vi "Handle Messages.vi"(8 "error in (no error)":errorcluster, 9 "Message Data":variant, 10 "Message":string, 11 "Coffee Shop In":refnum<class "Coffee Shop.lvclass">) -> (0 "error out":errorcluster, 3 "Coffee Shop Out":refnum<class "Coffee Shop.lvclass">)   [LabVIEW 2020, in "Coffee Shop.lvclass"]
uses:
  Coffee Shop.lvclass
  C:/Program Files (x86)/National Instruments/LabVIEW 2020/vi.lib/Asteme/Triarc Framework/Application/Application.lvclass
  C:/Program Files (x86)/National Instruments/LabVIEW 2020/vi.lib/Asteme/Triarc Framework/Process/Process.lvclass
  Customer/Customer.lvclass
  Public/Roles.ctl
  <vilib>/Asteme/Triarc Framework/Process/Process.lvclass/Process.ctl
  <vilib>/Asteme/Triarc Framework/Application/Application.lvclass/Application.ctl
  Coffee Shop.lvclass/Coffee Shop.ctl
  Process Job/Job Handler.lvclass
  <vilib>/Asteme/Triarc Framework/Application/Private/Add Process to Map.vi
  <vilib>/Asteme/Triarc Framework/Application/Private/Start Idle Processes if Running.vi
  <vilib>/Asteme/Triarc Framework/Process/Protected/Messaging/Enqueue Message.vi
  <vilib>/Asteme/Triarc Framework/Process/Protected/SubVIs/Set Context.vi
  <vilib>/Asteme/Triarc Framework/Process/Public/Lifecycle/Get Lifecycle State.vi
  <vilib>/Asteme/Triarc Framework/Process/Stop.vi
  <vilib>/Utility/error.llb/Clear Errors.vi
  <vilib>/Asteme/Triarc Framework/Process/Community/Leave Process Loop.vi
  <vilib>/Asteme/Triarc Framework/Process/Private/SubVIs/Wait for finish.vi
  <vilib>/Asteme/Triarc Framework/Process/Private/SubVIs/Set Lifecycle State.vi
  <vilib>/Asteme/Triarc Framework/Application/Application.lvclass
  <vilib>/Utility/error.llb/Error Cluster From Error Code.vi
  <vilib>/Asteme/Triarc Framework/Process/Start.vi
  <vilib>/Asteme/Triarc Framework/Application/Private/Update Context for Owned Processes.vi
  <vilib>/Asteme/Triarc Framework/Process/Process.lvclass
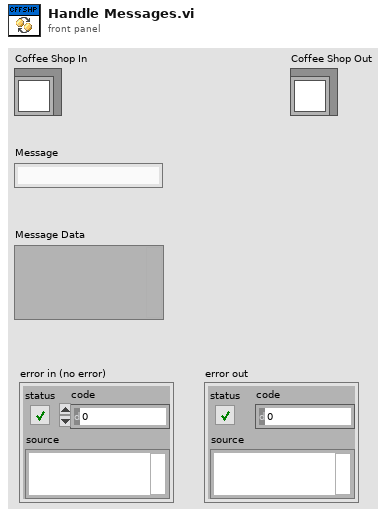
[diagram p1: front panel]
types:
  T1 = typedef "Coffee Shop.lvclass/Roles.ctl" = enum16{"Customer", "Barista", "Cashier"}
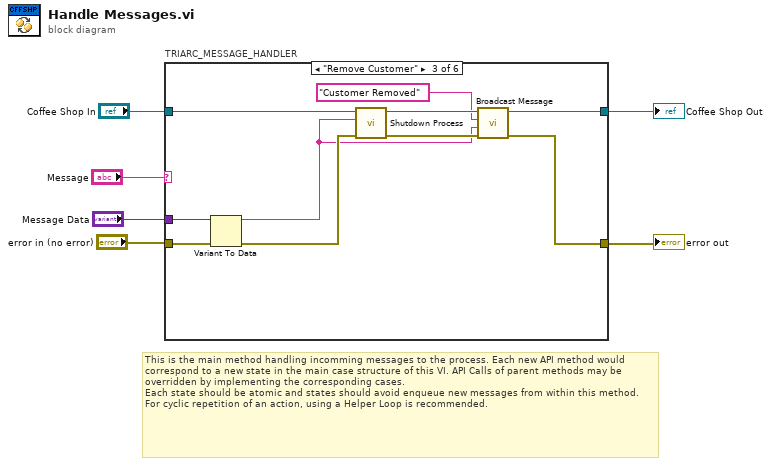
[diagram p0: block diagram]
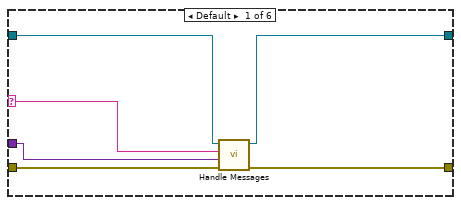
[diagram p2: hidden frame]
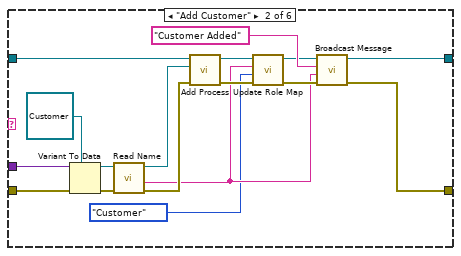
[diagram p3: hidden frame]
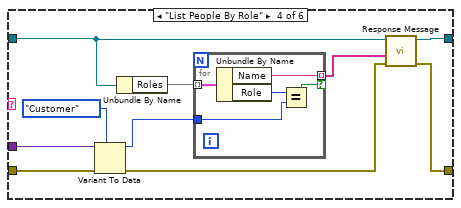
[diagram p4: hidden frame]
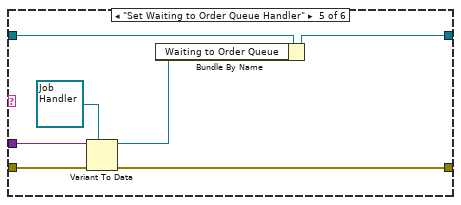
[diagram p5: hidden frame]
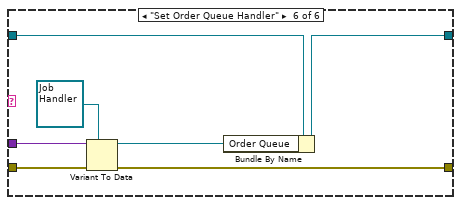
[diagram p6: hidden frame]
diagram:
  # "This is the main method handling incomming messages to the process. Each new API method would correspond to a new state in the main case structure of this VI. API Calls of parent methods may be overridden by implementing the corresponding cases.\nEach state should be atomic and states should avoid enqueue new messages from within this method. For cyclic repetition of an action, using a Helper Loop is recommended."
  n1 = case "TRIARC_MESSAGE_HANDLER" shown="\"Remove Customer\"" "Message" {
    selector: "Message" -> [w10 _ _ _ _ _]
    tunnel: "error in (no error)" -> [w9 w28 w39 w49 w61 w68]
    tunnel: "Coffee Shop In" -> [w12 w26 w37 w41 w60 w67]
    tunnel: "Message Data" -> [w11 w29 w38 w47 w57 w64]
    tunnel: [w8 w23 w34 w43 w59 w66] -> w2
    tunnel: [w7 w22 w32 w42 w56 w63] -> w1
    frame Default {
      n2 = call-parent "Handle Messages.vi"("error in (no error)"=w9, "Message Data"=w11, "Message"=w10, "Application In"=w12) -> ("error out"=w8:errorcluster, "Application Out"=w7:refnum<class "Coffee Shop.lvclass">)  [unwired: 6 in]
    }
    frame "Add Customer" {
      n3 = Variant To Data(error in=w28, type=refnum<class "Customer.lvclass"> refnum ("Customer.lvclass"), Variant=w29) -> (data=w19:refnum<class "Customer.lvclass">, error out=w25:errorcluster)
      n4 = call-dynamic "Read Name.vi"("error in (no error)"=w25, "Process In"=w19) -> ("error out"=w20:errorcluster, "Name"=w14:string, "Process Out"=w18:refnum<class "Customer.lvclass">)  [unwired: 6 in, 1 out]
      n5 = call <vilib>:"Add Process.vi"("error in (no error)"=w20, "Process"=w18, "Rig In"=w26) -> ("error out"=w24:errorcluster, "Rig Out"=w16:refnum<class "Coffee Shop.lvclass">)  [unwired: 7 in]
      n6 = call "Update Role Map.vi"("error in (no error)"=w24, "Role"=Roles."Customer", "Name"=w14, "Coffee Shop In"=w16) -> ("error out"=w17:errorcluster, "Coffee Shop Out"=w15:refnum<class "Coffee Shop.lvclass">)  [unwired: 6 in]
      n7 = call-dynamic "Broadcast Message.vi"("error in (no error)"=w17, "Message Data"=w14, "Message"="Customer Added", "Rig Process In"=w15) -> ("error out"=w23:errorcluster, "Rig Process Out"=w22:refnum<class "Coffee Shop.lvclass">)  [unwired: 6 in]
    }
    frame "Remove Customer" {
      n8 = Variant To Data(error in=w39, Variant=w38) -> (data=w30:string, error out=w36:errorcluster)  [unwired: 1 in]
      n9 = call <vilib>:"Shutdown Process.vi"("error in (no error)"=w36, "Process Name"=w30, "Rig In"=w37) -> ("error out"=w35:errorcluster, "Rig Out"=w33:refnum<class "Coffee Shop.lvclass">)  [unwired: 7 in]
      n10 = call-dynamic "Broadcast Message.vi"("error in (no error)"=w35, "Message Data"=w30, "Message"="Customer Removed", "Rig Process In"=w33) -> ("error out"=w34:errorcluster, "Rig Process Out"=w32:refnum<class "Coffee Shop.lvclass">)  [unwired: 6 in]
    }
    frame "List People By Role" {
      n11 = Variant To Data(error in=w49, type=Roles."Customer" ("Roles"), Variant=w47) -> (data=w44:T1, error out=w48:errorcluster)
      n12 = Unbundle By Name(w41) -> ("Roles"=w45:map{string, T1})
      n13 = for {
        tunnel: w45 -> [w54] mode=indexing
        tunnel: w44 -> [w50]
        tunnel: [w53] -> w40 mode=indexing if=w52
        n14 = Unbundle By Name(w54) -> ("Name"=w53:string, "Role"=w51:T1)
        n15 = Equal?(x=w51, y=w50) -> (x = y?=w52:bool)
      }
      n16 = call <vilib>:"Response Message.vi"("error in (no error)"=w48, "Response Message Data"=w40, "Process In"=w41) -> ("error out"=w43:errorcluster, "Process Out"=w42:refnum<class "Coffee Shop.lvclass">)  [unwired: 7 in]
    }
    frame "Set Waiting to Order Queue Handler" {
      n17 = Variant To Data(error in=w61, type=refnum<class "Job Handler.lvclass"> refnum ("Job Handler.lvclass"), Variant=w57) -> (data=w55:refnum<class "Job Handler.lvclass">, error out=w59:errorcluster)
      n18 = Bundle By Name(cluster=w60, "Waiting to Order Queue"=w55) -> (w56:refnum<class "Coffee Shop.lvclass">)
    }
    frame "Set Order Queue Handler" {
      n19 = Variant To Data(error in=w68, type=refnum<class "Job Handler.lvclass"> refnum ("Job Handler.lvclass"), Variant=w64) -> (data=w62:refnum<class "Job Handler.lvclass">, error out=w66:errorcluster)
      n20 = Bundle By Name(cluster=w67, "Order Queue"=w62) -> (w63:refnum<class "Coffee Shop.lvclass">)
    }
  }
  "error out" <- w2
  "Coffee Shop Out" <- w1
